vi "Sample Out.vi"(8 "error in (no error)":errorcluster, 11 "Preparation Line in":refnum<class "Preparation Line.lvclass">) -> (0 "error out":errorcluster, 3 "Preparation Line out":refnum<class "Preparation Line.lvclass">)   [LabVIEW 2015, in "cRIO-Carbondioxide.lvlib" / "CO2-Actor.lvlib" / "Preparation Line.lvclass"]
uses:
  Preparation Line.lvclass
  Valve/Valve.lvclass
  Preparation Line.lvclass/Preparation Line.ctl
  CO2 Actor Messages/Ping Msg/Ping Msg.lvclass/Ping Msg.ctl
  <vilib>/ActorFramework/Message Enqueuer/Message Enqueuer.lvclass/Message Enqueuer.ctl
  <vilib>/ActorFramework/Message Enqueuer/Enqueue.vi
  <vilib>/ActorFramework/Message Priority Queue/Priority Enqueue.vi
  CO2 Actor/CO2 Actor.lvclass
  CO2 Actor Messages/Ping Msg/Ping Msg.lvclass
  <vilib>/ActorFramework/Actor/Actor.lvclass
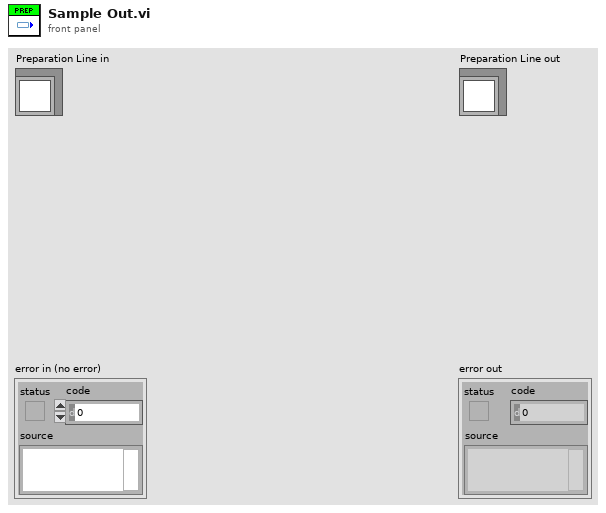
[diagram p1: front panel]
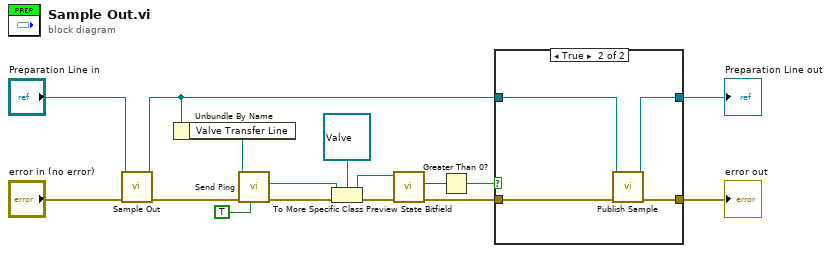
[diagram p0: block diagram]
diagram:
  n1 = call-parent "Sample Out.vi"("error in (no error)"="error in (no error)", "CO2 Actor in"="Preparation Line in") -> ("error out"=w14:errorcluster, "CO2 Actor out"=w4:refnum<class "Preparation Line.lvclass">)  [unwired: 8 in]
  n2 = Unbundle By Name(w4) -> ("Valve Transfer Line"=w12:refnum<class "Message Enqueuer.lvclass">)
  n3 = call "Send Ping.vi"("Return Self (F)"=TRUE, "error in (no error)"=w14, "Message Enqueuer"=w12) -> ("error out"=w7:errorcluster, "Actor out"=w6:refnum<class "Actor.lvclass">)  [unwired: 5 in, 2 out]
  n4 = To More Specific Class(target class=refnum<class "Valve.lvclass"> refnum ("Valve.lvclass"), reference=w6, error in=w7) -> (specific class reference=w10:refnum<class "Valve.lvclass">, error out=w9:errorcluster)
  n5 = call "Preview State Bitfield.vi"("error in (no error)"=w9, "Valve in"=w10) -> ("error out"=w5:errorcluster, "State Bitfield"=w11:u16)  [unwired: 7 in, 1 out]
  n6 = Greater Than 0?(x=w11) -> (x > 0?=w1:bool)
  n7 = case shown="True" w1 {
    tunnel: w5 -> [w17 w19]
    tunnel: w4 -> [w18 w20]
    tunnel: [w18 w22] -> w3
    tunnel: [w17 w21] -> w2
    frame False {
    }
    frame True {
      n8 = call "Publish Sample.vi"("error in (no error)"=w19, "Preparation Line in"=w20) -> ("error out"=w21:errorcluster, "Preparation Line out"=w22:refnum<class "Preparation Line.lvclass">)  [unwired: 8 in]
    }
  }
  "error out" <- w2
  "Preparation Line out" <- w3
